vi "FGV_Undo Redo.vi"(7 "Action":T8, 8 "error in (no error)":errorcluster, 10 "Data in":string, 11 "Data in":T1={"Class"={"Ants"=refnum, "Layer"=refnum, "Templates"=refnum, "Icon"=refnum, "Glyph"=refnum, "Settings"=refnum, "Tools"=refnum}, "Ref"={"Add Layer"=refnum, "Remove Layer"=refnum, "Line Text"=[], "Body Text Spec"=refnum, "DNL_Font"=refnum, "glyph path str"=refnum, "templates path str"=refnum, "Arrow Up"=refnum, "Arrow Down"=refnum, "IE VI Ref"=refnum, "Glyphs tree"=refnum, "Templates tree"=refnum, "Layer Icon Text"=refnum, "Layer Template"=refnum, "Clipboard"=refnum, "BW icon in"=refnum, "Color icon in"=refnum, "Layer Clust"=refnum, "Body Text"=refnum, "DNL_Framework Templates"=refnum, "Search Templates"=refnum, "TextMarker"=refnum, "Tab Control"=refnum, "Search Glyphs"=refnum, "Line Color"=refnum, "DNL_Glyphs []"=refnum, "Fill Color"=refnum, "Tools"=refnum, "Glyphs tree"=refnum, "Icon"=refnum, "Preview"=refnum, "Ants"=refnum, "Terminals"=refnum, "menu reference"=refnum, "LayerNames"=[], "GlyphLoadAnimation"=refnum, "TemplateLoadAnimation"=refnum, "refreshGlyphs"=refnum, "refreshTemplates"=refnum}, "Support"={"AntsRect"={"left"=0, "top"=0, "right"=0, "bottom"=0}, "Mouse Move Coords"={"Horizontal"=0, "Vertical"=0}, "Mouse Down Coords"={"Horizontal"=0, "Vertical"=0}, "Temp Coord"={"Horizontal"=0, "Vertical"=0}, "Action"=enum."Default", "Edge Color"=4914962, "Fill Color"=16860, "Mouse Down?"=FALSE, "Draft Mode?"=FALSE, "Temp Icon"=bytes[3102], "CTRL Pressed"=FALSE, "Move Selection?"=FALSE, "AntsRect Orig"={"left"=0, "top"=0, "right"=0, "bottom"=0}, "Text"="", "TM Set?"=FALSE, "Mouse inside icon?"=FALSE, "Tool (old value)"=0, "Pencil Move Color"=0, "Swap Colors?"=FALSE, "Shift pressed?"=FALSE}}) -> (0 "error out":errorcluster, 2 "Data out":string, 3 "Data out":T1={"Class"={"Ants"=refnum, "Layer"=refnum, "Templates"=refnum, "Icon"=refnum, "Glyph"=refnum, "Settings"=refnum, "Tools"=refnum}, "Ref"={"Add Layer"=refnum, "Remove Layer"=refnum, "Line Text"=[], "Body Text Spec"=refnum, "DNL_Font"=refnum, "glyph path str"=refnum, "templates path str"=refnum, "Arrow Up"=refnum, "Arrow Down"=refnum, "IE VI Ref"=refnum, "Glyphs tree"=refnum, "Templates tree"=refnum, "Layer Icon Text"=refnum, "Layer Template"=refnum, "Clipboard"=refnum, "BW icon in"=refnum, "Color icon in"=refnum, "Layer Clust"=refnum, "Body Text"=refnum, "DNL_Framework Templates"=refnum, "Search Templates"=refnum, "TextMarker"=refnum, "Tab Control"=refnum, "Search Glyphs"=refnum, "Line Color"=refnum, "DNL_Glyphs []"=refnum, "Fill Color"=refnum, "Tools"=refnum, "Glyphs tree"=refnum, "Icon"=refnum, "Preview"=refnum, "Ants"=refnum, "Terminals"=refnum, "menu reference"=refnum, "LayerNames"=[], "GlyphLoadAnimation"=refnum, "TemplateLoadAnimation"=refnum, "refreshGlyphs"=refnum, "refreshTemplates"=refnum}, "Support"={"AntsRect"={"left"=0, "top"=0, "right"=0, "bottom"=0}, "Mouse Move Coords"={"Horizontal"=0, "Vertical"=0}, "Mouse Down Coords"={"Horizontal"=0, "Vertical"=0}, "Temp Coord"={"Horizontal"=0, "Vertical"=0}, "Action"=enum."Default", "Edge Color"=4914962, "Fill Color"=16860, "Mouse Down?"=FALSE, "Draft Mode?"=FALSE, "Temp Icon"=bytes[3102], "CTRL Pressed"=FALSE, "Move Selection?"=FALSE, "AntsRect Orig"={"left"=0, "top"=0, "right"=0, "bottom"=0}, "Text"="", "TM Set?"=FALSE, "Mouse inside icon?"=FALSE, "Tool (old value)"=0, "Pencil Move Color"=0, "Swap Colors?"=FALSE, "Shift pressed?"=FALSE}})   [LabVIEW 2021]
uses:
  <resource>/plugins/NIIconEditor/Controls/Undo Redo Action.ctl
  <resource>/plugins/NIIconEditor/Controls/IE Data.ctl
  <resource>/plugins/NIIconEditor/Class/Ants/Ants.lvclass
  <resource>/plugins/NIIconEditor/Class/FakedArray/FakedArray.lvclass
  <resource>/plugins/NIIconEditor/Class/Icon Library/Glyph.lvclass
  <resource>/plugins/NIIconEditor/Class/Settings/Settings.lvclass
  <resource>/plugins/NIIconEditor/Class/Tools/Tools Paint.lvclass
  <vilib>/LabVIEW Icon API/lv_icon/Classes/Icon/Icon.lvclass
  <resource>/plugins/NIIconEditor/Controls/IE Classes.ctl
  <resource>/plugins/NIIconEditor/Controls/References Cluster.ctl
  <resource>/plugins/NIIconEditor/Controls/SupportClass.ctl
  <vilib>/Utility/miscctls.llb/LVPoint32TypeDef.ctl
  <resource>/plugins/NIIconEditor/Controls/SupportClass_Action.ctl
  <vilib>/LabVIEW Icon API/lv_icon/Controls/IEColor.ctl
  <resource>/dialog/lvconfig.llb/LV Config Read Color.vi
panel:
  out "# valid elements":i32
  out "undo":i32
  out "curr pointer":i32
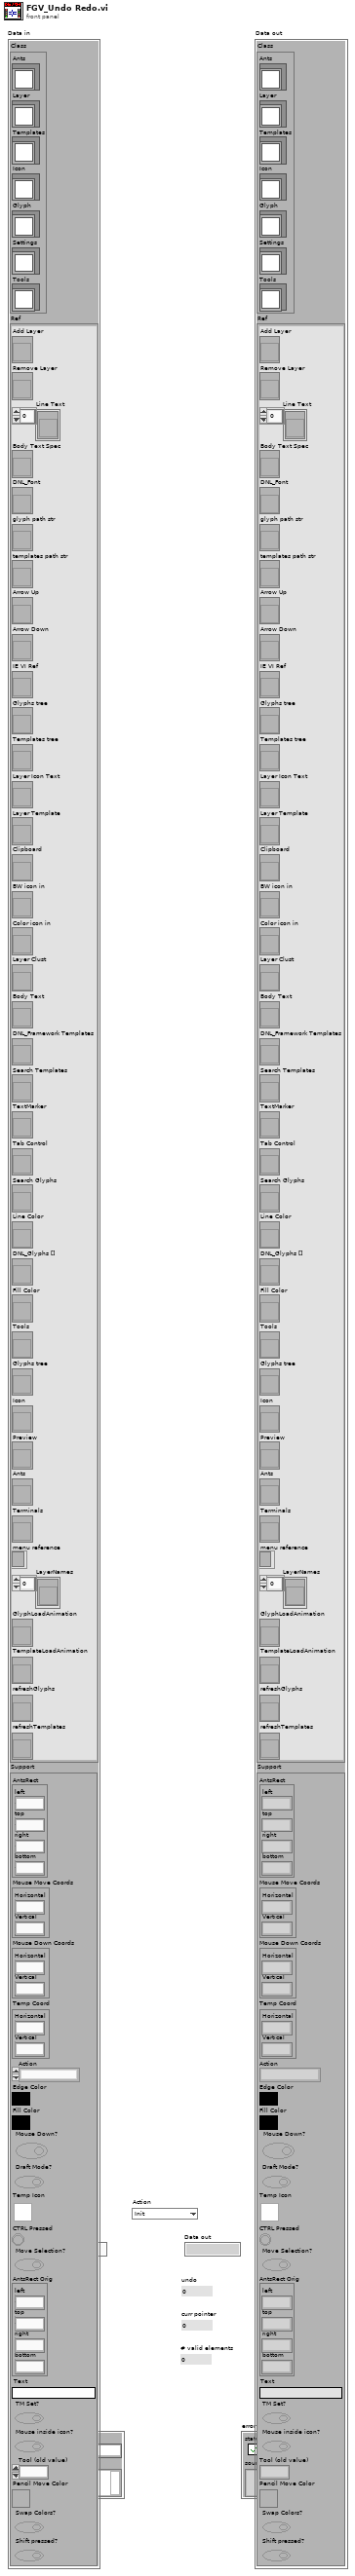
[diagram p1: front panel]
types:
  T1 = typedef "IE Data.ctl" = cluster{"Class":T2, "Ref":T3, "Support":T4}
  T2 = typedef "IE Classes.ctl" = cluster{"Ants":refnum<class "Ants.lvclass">, "Layer":refnum<class "FakedArray.lvclass">, "Templates":refnum<class "FakedArray.lvclass">, "Icon":refnum<class "Icon.lvclass">, "Glyph":refnum<class "Glyph.lvclass">, "Settings":refnum<class "Settings.lvclass">, "Tools":refnum<class "Tools Paint.lvclass">}
  T3 = typedef "References Cluster.ctl" = cluster{"Add Layer":refnum<vi>, "Remove Layer":refnum<vi>, "Line Text":refnum<vi>[], "Body Text Spec":refnum<vi>, "DNL_Font":refnum<vi>, "glyph path str":refnum<vi>, "templates path str":refnum<vi>, "Arrow Up":refnum<vi>, "Arrow Down":refnum<vi>, "IE VI Ref":refnum<vi>, "Glyphs tree":refnum<vi>, "Templates tree":refnum<vi>, "Layer Icon Text":refnum<vi>, "Layer Template":refnum<vi>, "Clipboard":refnum<vi>, "BW icon in":refnum<vi>, "Color icon in":refnum<vi>, "Layer Clust":refnum<vi>, "Body Text":refnum<vi>, "DNL_Framework Templates":refnum<vi>, "Search Templates":refnum<vi>, "TextMarker":refnum<vi>, "Tab Control":refnum<vi>, "Search Glyphs":refnum<vi>, "Line Color":refnum<vi>, "DNL_Glyphs []":refnum<vi>, "Fill Color":refnum<vi>, "Tools":refnum<vi>, "Glyphs tree":refnum<vi>, "Icon":refnum<vi>, "Preview":refnum<vi>, "Ants":refnum<vi>, "Terminals":refnum<vi>, "menu reference":refnum<k9>, "LayerNames":refnum<vi>[], "GlyphLoadAnimation":refnum<vi>, "TemplateLoadAnimation":refnum<vi>, "refreshGlyphs":refnum<vi>, "refreshTemplates":refnum<vi>}
  T4 = typedef "SupportClass.ctl" = cluster{"AntsRect":cluster{"left":i16, "top":i16, "right":i16, "bottom":i16}, "Mouse Move Coords":T5, "Mouse Down Coords":T5, "Temp Coord":T5, "Action":T6, "Edge Color":T7, "Fill Color":T7, "Mouse Down?":bool, "Draft Mode?":bool, "Temp Icon":picture, "CTRL Pressed":bool, "Move Selection?":bool, "AntsRect Orig":cluster{"left":i16, "top":i16, "right":i16, "bottom":i16}, "Text":string, "TM Set?":bool, "Mouse inside icon?":bool, "Tool (old value)":u32, "Pencil Move Color":u32, "Swap Colors?":bool, "Shift pressed?":bool}
  T5 = typedef "LVPoint32TypeDef.ctl" = cluster{"Horizontal":i32, "Vertical":i32}
  T6 = typedef "SupportClass_Action.ctl" = enum16{"Default", "Move Selection", "Glyph Library", "Tool"}
  T7 = typedef "IEColor.ctl" = u32
  T8 = typedef "Undo Redo Action.ctl" = enum16{"Init", "Add", "Redo", "Undo", "Undo Preview"}
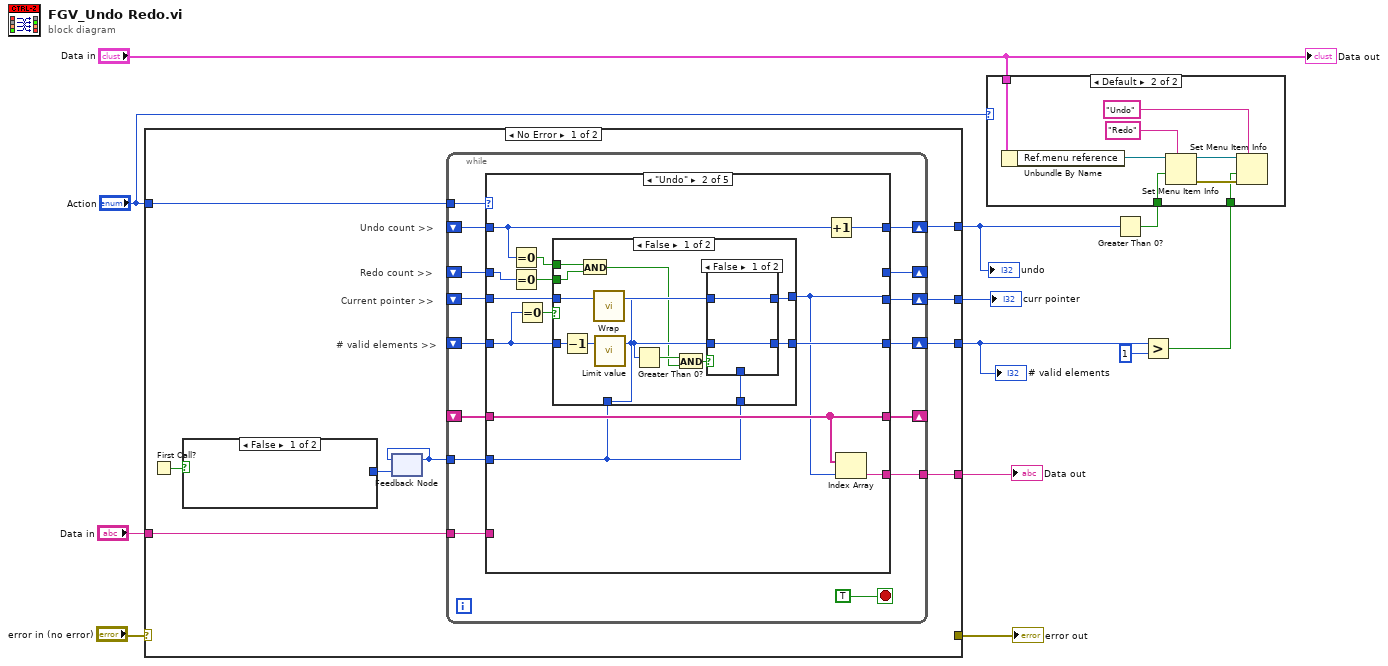
[diagram p0: block diagram]
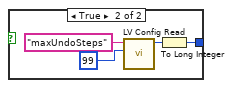
[diagram p3: hidden frame]
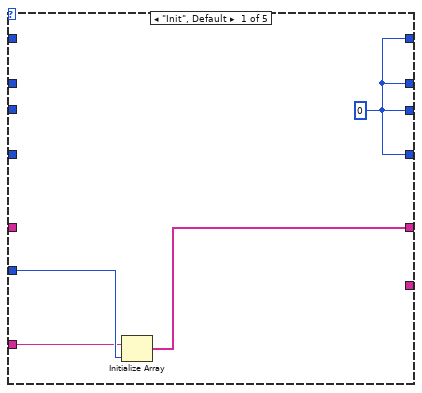
[diagram p4: hidden frame]
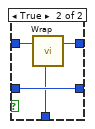
[diagram p5: hidden frame]
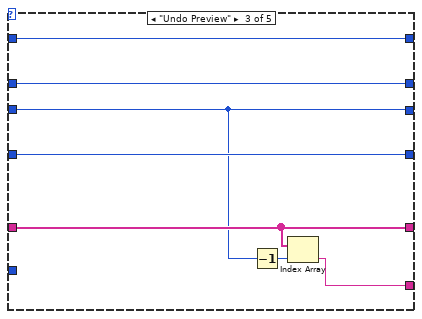
[diagram p7: hidden frame]
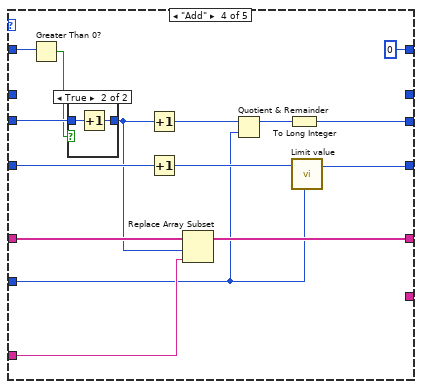
[diagram p8: hidden frame]
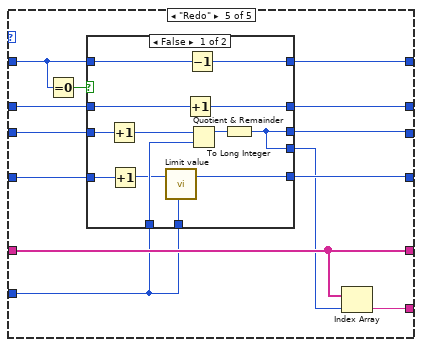
[diagram p10: hidden frame]
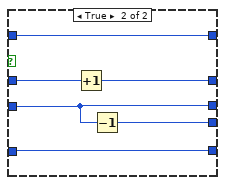
[diagram p11: hidden frame]
diagram:
  n1 = case shown="No Error" "error in (no error)" {
    selector: "error in (no error)" -> [_ w137]
    tunnel: [_ w137] -> w11
    tunnel: "Action" -> [w21 _]
    tunnel: "Data in" -> [w20 _]
    tunnel: [w19 _] -> w7
    tunnel: [w18 _] -> w1
    tunnel: [w15 _] -> w8
    tunnel: [w14 _] -> w6
    frame No Error {
      # "Redo count >>"
      # "# valid elements >>"
      # "Undo count >>"
      # "Current pointer >>"
      n2 = First Call?() -> (First Call?: T/F=w17:bool)
      n3 = case shown="False" w17 {
        tunnel: [_ w22] -> w13
        frame False {
        }
        frame True {
          n4 = call-poly <resource>:"LV Config Read.vi"("default value"=99, "key"="maxUndoSteps") -> ("value"=w23:u32)  [unwired: 1 in, 4 out]
          n5 = To Long Integer(number=w23) -> (32bit integer=w22:i32)
        }
      }
      n6 = feedback #1(w13) -> (w16:i32)
      n7 = feedback-in #1(w16) -> ()
      n8 = while {
        tunnel: w21 -> [w39]
        shift-right: [w38] -> _
        shift-left: _ -> [w37]
        tunnel: w20 -> [w36]
        shift-right: [w35] -> w14
        shift-left: _ -> [w34]
        shift-right: [w32] -> w15
        shift-left: _ -> [w33]
        shift-right: [w30] -> w18
        shift-left: _ -> [w31]
        tunnel: [w29] -> w19
        tunnel: w16 -> [w28]
        shift-right: [w26] -> _
        shift-left: _ -> [w27]
        stop <- TRUE stop-if-true
        n9 = case shown="\"Undo\"" w39 {
          tunnel: [w44 w55 w84 w101 w116] -> w38
          tunnel: w37 -> [_ w55 w84 w95 w116]
          tunnel: w36 -> [w42 _ _ w91 _]
          tunnel: [w41 w53 w82 w97 w110] -> w35
          tunnel: w34 -> [_ w57 w82 w99 w114]
          tunnel: w33 -> [_ w48 w86 w88 w108]
          tunnel: [w41 w50 w86 0 w117] -> w32
          tunnel: w31 -> [_ w51 w85 w96 w113]
          tunnel: [w41 w56 w85 w93 w112] -> w30
          tunnel: [_ w54 w81 _ w115] -> w29
          tunnel: w28 -> [w43 w49 _ w89 w107]
          tunnel: w27 -> [_ w46 w80 _ w106]
          tunnel: [w41 _ w80 _ w105] -> w26
          frame "Init", Default {
            w41 = 0
            n10 = Initialize Array(w42, w43) -> (w44:string[])
          }
          frame "Undo" {
            n11 = Equal To 0?(x=w48) -> (x = 0?=w47:bool)
            n12 = Equal To 0?(x=w46) -> (x = 0?=w45:bool)
            n13 = Equal To 0?(x=w51) -> (x = 0?=w52:bool)
            n14 = case shown="False" w52 {
              tunnel: w57 -> [w69 w79]
              tunnel: w51 -> [w71 w78]
              tunnel: [w64 w78] -> w56
              tunnel: [w65 w79] -> w53
              tunnel: w49 -> [w62 _]
              tunnel: w49 -> [w61 _]
              tunnel: w47 -> [w60 _]
              tunnel: w45 -> [w59 _]
              frame False {
                n15 = Decrement(x=w71) -> (x-1=w70:i32)
                n16 = And(x=w60, y=w59) -> (x .and. y?=w58:bool)
                n17 = call <resource>:"Wrap.vi"("Current Value in"=w69, "max undo steps"=w62) -> ("Value out"=w68:i32)  [unwired: 17 out]
                n18 = call <resource>:"Limit value.vi"("Current Value in"=w70, "max undo steps"=w62) -> ("Value out"=w67:i32)  [unwired: 1 in, 16 out]
                n19 = Greater Than 0?(x=w67) -> (x > 0?=w63:bool)
                n20 = And(x=w63, y=w58) -> (x .and. y?=w66:bool)
                n21 = case shown="False" w66 {
                  tunnel: w67 -> [w72 w75]
                  tunnel: w68 -> [w73 w77]
                  tunnel: [w73 w76] -> w65
                  tunnel: [w72 w75] -> w64
                  tunnel: w61 -> [_ w74]
                  frame False {
                  }
                  frame True {
                    n22 = call <resource>:"Wrap.vi"("Current Value in"=w77, "max undo steps"=w74) -> ("Value out"=w76:i32)  [unwired: 17 out]
                  }
                }
              }
              frame True {
              }
            }
            n23 = Increment(x=w48) -> (x+1=w50:i32)
            n24 = Index Array(array=w55, index=w53) -> (element=w54:string)
          }
          frame "Undo Preview" {
            n25 = Decrement(x=w82) -> (x-1=w83:i32)
            n26 = Index Array(array=w84, index=w83) -> (element=w81:string)
          }
          frame "Add" {
            n27 = Greater Than 0?(x=w88) -> (x > 0?=w87:bool)
            n28 = case shown="True" w87 {
              tunnel: w99 -> [w102 w104]
              tunnel: [w102 w103] -> w90
              frame False {
              }
              frame True {
                n29 = Increment(x=w104) -> (x+1=w103:i32)
              }
            }
            n30 = Increment(x=w90) -> (x+1=w100:i32)
            n31 = Increment(x=w96) -> (x+1=w94:i32)
            n32 = Replace Array Subset(array=w95, new element=w91, index=w90) -> (w101:string[])
            n33 = Quotient & Remainder(x=w100, y=w89) -> (x-y*floor(x/y)=w98:i32)  [unwired: 1 out]
            n34 = To Long Integer(number=w98) -> (32bit integer=w97:i32)
            n35 = call <resource>:"Limit value.vi"("Current Value in"=w94, "max undo steps"=w89) -> ("Value out"=w93:i32)  [unwired: 1 in, 16 out]
          }
          frame "Redo" {
            n36 = Equal To 0?(x=w108) -> (x = 0?=w111:bool)
            n37 = case shown="False" w111 {
              tunnel: w108 -> [w130 w136]
              tunnel: [w129 w136] -> w117
              tunnel: w114 -> [w128 w134]
              tunnel: w113 -> [w127 w135]
              tunnel: w107 -> [w122 _]
              tunnel: [w123 w135] -> w112
              tunnel: [w124 w134] -> w110
              tunnel: [w124 w133] -> w109
              tunnel: w107 -> [w120 _]
              tunnel: w106 -> [w119 w132]
              tunnel: [w118 w131] -> w105
              frame False {
                n38 = Increment(x=w128) -> (x+1=w125:i32)
                n39 = Increment(x=w127) -> (x+1=w121:i32)
                n40 = call <resource>:"Limit value.vi"("Current Value in"=w121, "max undo steps"=w120) -> ("Value out"=w123:i32)  [unwired: 1 in, 16 out]
                n41 = Increment(x=w119) -> (x+1=w118:i32)
                n42 = Decrement(x=w130) -> (x-1=w129:i32)
                n43 = Quotient & Remainder(x=w125, y=w122) -> (x-y*floor(x/y)=w126:i32)  [unwired: 1 out]
                n44 = To Long Integer(number=w126) -> (32bit integer=w124:i32)
              }
              frame True {
                n45 = Increment(x=w132) -> (x+1=w131:i32)
                n46 = Decrement(x=w134) -> (x-1=w133:i32)
              }
            }
            n47 = Index Array(array=w116, index=w109) -> (element=w115:string)
          }
        }
      }
    }
    frame Error {
    }
  }
  "error out" <- w11
  "Data out" <- w7
  "curr pointer" <- w6
  "undo" <- w8
  "# valid elements" <- w1
  n48 = Greater Than 0?(x=w8) -> (x > 0?=w9:bool)
  n49 = Greater?(x=w1, y=1) -> (0:w4:bool)
  n50 = case shown="Default" "Action" {
    tunnel: w9 -> [_ w141]
    tunnel: "Data in" -> [_ w140]
    tunnel: w4 -> [_ w138]
    frame "Undo Preview" {
    }
    frame Default {
      n51 = Unbundle By Name(w140) -> ("Ref.menu reference"=w139:refnum<k9>)
      n52 = Set Menu Item Info(7:"Redo" ("Redo Menu Item"), 9:w141, 11:w139) -> (0:w145:errorcluster, 3:w144:refnum<k9>)  [unwired: 1 in, 3 out]
      n53 = Set Menu Item Info(7:"Undo" ("Undo Menu Item"), 8:w145, 9:w138, 11:w144) -> ()  [unwired: 5 out]
    }
  }
  "Data out" <- "Data in"
